vi "PmodTMP3open.vi"(7 "I2C Channel (0)":u8, 8 "error in (no error)":errorcluster, 9 "Resolution":enum16{"0.5", "0.25", "0.125", "0.0625"}(ring), 10 "Slave Address":T7(ring), 11 "LINX Ref":T1) -> (0 "error out":errorcluster, 1 "Resolution":enum16{"0.5", "0.25", "0.125", "0.0625"}(ring), 3 "LINX Resource":T1)   [LabVIEW 2014]
doc: "Open communication to the PmodTMP3 and set the desired resolution in the 0x01 register."
uses:
  <vilib>/MakerHub/LINX/Private/Type Defs/LINX Ref.ctl
  <vilib>/MakerHub/LINX/Private/Type Defs/Platform.ctl
  <vilib>/MakerHub/LINX/Private/Type Defs/Interface.ctl
  <vilib>/MakerHub/LINX/Private/Device/Type Defs/LINX Device Config.ctl
  <vilib>/MakerHub/LINX/Private/Device/Type Defs/TCP Config.ctl
  <vilib>/MakerHub/LINX/Private/Device/Type Defs/Channels.ctl
  <vilib>/MakerHub/LINX/LMH-LINX.lvlib
  <vilib>/MakerHub/LINX/Private/Device/Device.lvlib
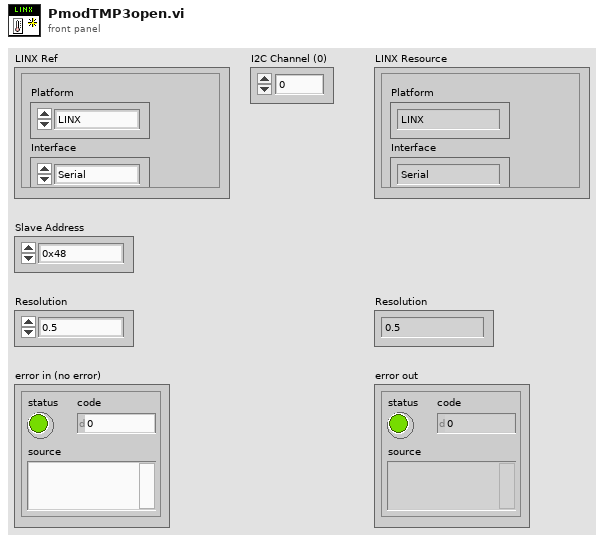
[diagram p1: front panel]
types:
  T1 = typedef "LMH-LINX.lvlib/LINX Ref.ctl" = cluster{"Platform":T2, "Interface":T3, "LINX Device Config":T4}
  T2 = typedef "LMH-LINX.lvlib/Platform.ctl" = enum16{"LINX", "myRIO"}
  T3 = typedef "LMH-LINX.lvlib/Interface.ctl" = enum16{"Serial", "TCP"}
  T4 = typedef "LMH-LINX.lvlib/Device.lvlib/LINX Device Config.ctl" = cluster{"Interface":T3, "COM Port":refnum<visa-resource-name>, "TCP Configuration":T5, "Device Family":u8, "Device ID":u8, "Device Name":string, "TCP Ref":refnum<k5>, "Channels":T6}
  T5 = typedef "LMH-LINX.lvlib/Device.lvlib/TCP Config.ctl" = cluster{"IP Address":string, "Port":u16}
  T6 = typedef "LMH-LINX.lvlib/Channels.ctl" = cluster{"DI":u8[], "DO":u8[], "AI":u8[], "AO":u8[], "PWM":u8[], "QE":u8[], "UART":u8[], "I2C 2":u8[], "SPI":u8[], "CAN":u8[], "Servo":u8[], "AI Ref (V)":dbl, "AO Ref (V)":dbl, "AO Resolution (Bits)":u8}
  T7 = enum8{"0x48", "0x49", "0x4A", "0x4B", "0x4C", "0x4D", "0x4E", "0x4F"}
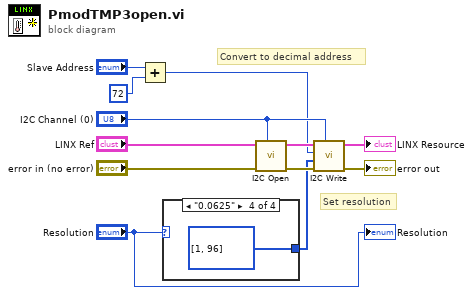
[diagram p0: block diagram]
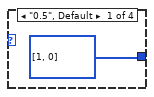
[diagram p2: hidden frame]
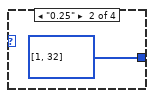
[diagram p3: hidden frame]
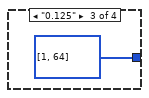
[diagram p4: hidden frame]
diagram:
  # "Set resolution"
  # "Convert to decimal address"
  n1 = Add(x="Slave Address", y=u8 72) -> (x+y=w1:u8)
  n2 = case shown="\"0.0625\"" "Resolution" {
    tunnel: [u8[] [1, 0] ("Data") u8[] [1, 32] ("Data") u8[] [1, 64] ("Data") u8[] [1, 96] ("Data")] -> w7
    frame "0.5", Default {
    }
    frame "0.25" {
    }
    frame "0.125" {
    }
    frame "0.0625" {
    }
  }
  n3 = call <vilib>:"I2C Open.vi"("I2C Channel (0)"="I2C Channel (0)", "Error In"="error in (no error)", "LINX Resource"="LINX Ref") -> ("Error Out"=w9:errorcluster, "LINX Resource"=w8:T1)  [unwired: 7 in]
  n4 = call <vilib>:"I2C Write.vi"("I2C Channel"="I2C Channel (0)", "Error In"=w9, "Data"=w7, "I2C Slave Address (0)"=w1, "LINX Resource"=w8) -> ("Error Out"=→"error out":errorcluster, "LINX Resource"=→"LINX Resource":T1)  [unwired: 5 in]
  "Resolution" <- "Resolution"
